vi "Axis Enum to String.vi"(8 "error in (no error)":errorcluster, 10 "Axis Enum In":T1=enum."A") -> (0 "error out":errorcluster, 2 "Axis String Out":string)   [LabVIEW 2018, in "ASI TG-1000.lvlib"]
uses:
  ASI TG-1000.lvlib
  Axis Name.ctl
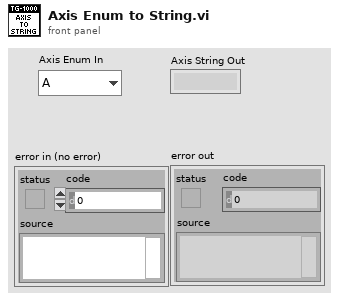
[diagram p1: front panel]
types:
  T1 = typedef "ASI TG-1000.lvlib/Axis Name.ctl" = enum8{"undefined", "A", "B", "C", "D", "E", "F", "G", "H", "I", "J", "K", "L", "M", "N", "O", "P", "Q", "R", "S", "T", "U", "V", "W", "X", "Y", "Z"}
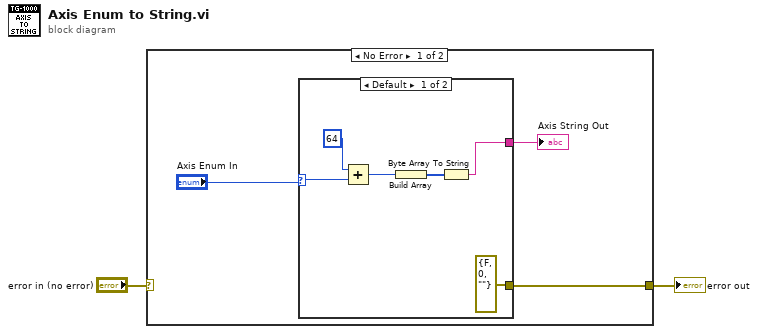
[diagram p0: block diagram]
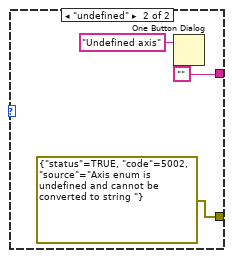
[diagram p2: hidden frame]
diagram:
  n1 = case shown="No Error" "error in (no error)" {
    selector: "error in (no error)" -> [_ w15]
    tunnel: [w4 w15] -> w1
    frame No Error {
      n2 = case shown="Default" "Axis Enum In" {
        selector: "Axis Enum In" -> [w10 _]
        tunnel: [errorcluster {"status"=FALSE, "code"=0, "source"=""} ("error constant") errorcluster {"status"=TRUE, "code"=5002, "source"="Axis enum is undefined and cannot be converted to string "} ("error constant")] -> w4
        tunnel: [w6 ""] -> w3
        frame Default {
          n3 = Add(x=64, y=w10) -> (x+y=w7:i32)
          n4 = Build Array(w7) -> (w8:i32[])
          n5 = Byte Array To String(unsigned byte array=w8) -> (string=w6:string)
        }
        frame "undefined" {
          n6 = One Button Dialog(message="Undefined axis") -> ()  [unwired: 1 in, 1 out]
        }
      }
      "Axis String Out" <- w3
    }
    frame Error {
    }
  }
  "error out" <- w1
